vi "Replace Multiple Items at Offsets.vi"(8 "error in (no error)":errorcluster, 9 "New JSON Items":string[](array[string]), 10 "Offsets of Items to Replace":i32[](array[numeric]), 11 "JSON":string) -> (0 "error out":errorcluster, 3 "<JSON>":string)   [LabVIEW 2019, in "JSONtext.lvlib"]
doc: "Replace the JSON Values located at Offsets in the input JSON. The Offsets can be that returned by a previous \"Find\" operation on the input JSON."
uses:
  JSONtext.lvlib
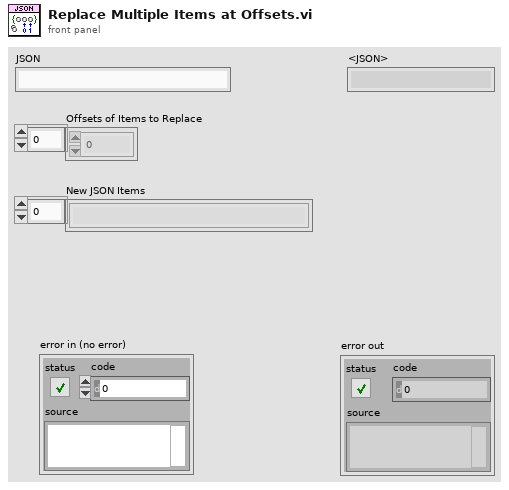
[diagram p1: front panel]
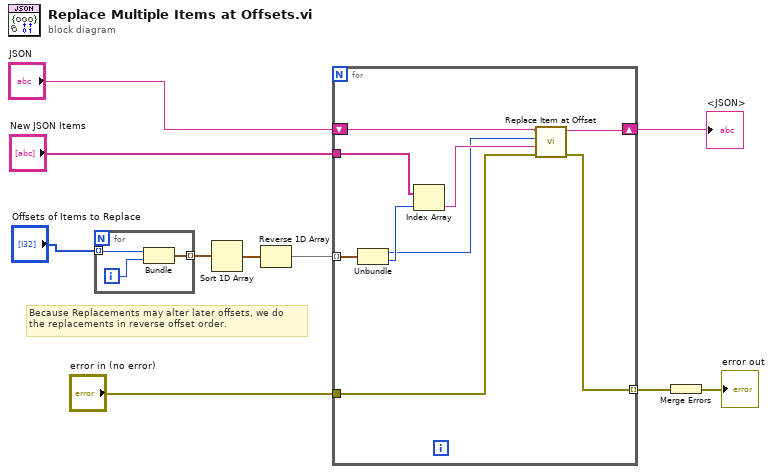
[diagram p0: block diagram]
diagram:
  # "Because Replacements may alter later offsets, we do \nthe replacements in reverse offset order."
  n1 = for {
    tunnel: "Offsets of Items to Replace" -> [w12] mode=indexing
    tunnel: [w11] -> w6 mode=indexing
    i -> [w13]
    n2 = Bundle("Offset of Item to Replace"=w12, w13) -> (w11:cluster{"Offset of Item to Replace":i32, i32})  [unwired: 1 in]
  }
  n3 = Sort 1D Array(array=w6) -> (sorted array=w5:cluster{"Offset of Item to Replace":i32, i32}[])
  n4 = Reverse 1D Array(array=w5) -> (reversed array=w4:cluster{"Offset of Item to Replace":i32, i32}[])
  n5 = for {
    tunnel: "New JSON Items" -> [w21]
    shift-right: [w18] -> w9
    shift-left: "JSON" -> [w19]
    tunnel: w4 -> [w22] mode=indexing
    tunnel: "error in (no error)" -> [w15]
    tunnel: [w14] -> w2 mode=indexing
    n6 = Unbundle(w22) -> ("Offset of Item to Replace"=w16:i32, w20:i32)
    n7 = Index Array(array=w21, index=w20) -> (element=w17:string)
    n8 = call "Replace Item at Offset.vi"("error in (no error)"=w15, "New JSON Item"=w17, "Offset of Item to Replace"=w16, "JSON"=w19) -> ("error out"=w14:errorcluster, "<JSON>"=w18:string)  [unwired: 6 in]
  }
  "<JSON>" <- w9
  n9 = Merge Errors(w2) -> (→"error out":errorcluster)
